vi "PlotDeviation.vi"(11 "Array":i32[][](array[numeric])) -> (0 "Deviation by row":dbl[][](array[numeric]) format="%.2f", 1 "Average in row":u64[](array[numeric]) format="%-2.0f", 2 "STD":dbl[](array[numeric]) format="%#_3g", 3 "Waveform Chart":i64[][](graph))   [LabVIEW 2023]
panel:
  out "Waveform Graph":dbl[][](graph)
  out "Table Control":string[][](table)
  out "2D Double Array":i32[][](array[numeric])
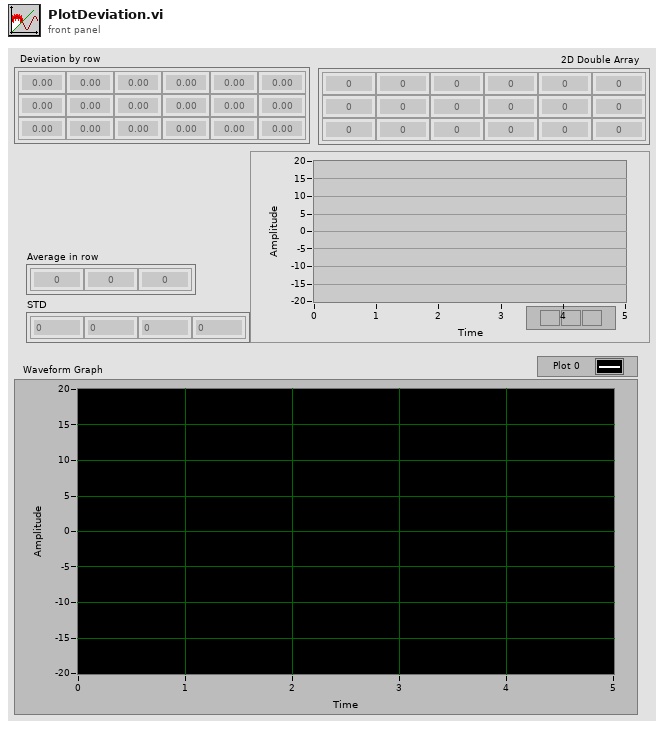
[diagram p1: front panel]
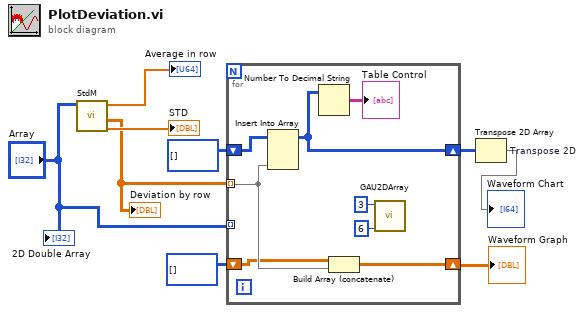
[diagram p0: block diagram]
diagram:
  n1 = call "StdM.vi"("2D in"="Array") -> ("1D Std"=→"STD":dbl[], "[Xi-X]"=w2:dbl[][], "Mean"=→"Average in row":dbl[])  [unwired: 6 in, 2 out]
  "Deviation by row" <- w2
  n2 = for {
    tunnel: w2 -> [w13] mode=indexing
    shift-right: [w15] -> w8
    shift-left: i64[][] [] -> [w17]
    tunnel: "Array" -> [_] mode=indexing
    shift-right: [w14] -> w5
    shift-left: i64[][] [] -> [w12]
    n3 = Insert Into Array "Insert Into Array"(array=w17, new element=w13) -> (w15:i64[][])  [unwired: 2 in]
    n4 = Number To Decimal String(number=w15) -> (decimal integer string=→"Table Control":string[][])  [unwired: 1 in]
    n5 = Build Array (concatenate)(w12, w13) -> (w14:dbl[][])
    n6 = call "GAU2DArray.vi"("Colums"=6, "Rows"=3) -> ()  [unwired: 7 in, 3 out]
  }
  "Waveform Graph" <- w5
  n7 = Transpose 2D Array "Transpose 2D"(2D array=w8) -> (transposed array=→"Waveform Chart":i64[][])
  "2D Double Array" <- "Array"
